vi "Acquisition Engine.vi"(0 "all channels":cluster{fxp<+/-,12,1>[]}[](array[cluster])=[{[0.0, 0.0, 0.0, 0.0, 0.0, 0.0, 0.0, 0.0, 0.0, 0.0, 0.0, 0.0, 0.0, 0.0, 0.0, 0.0]}, {[0.0, 0.0, 0.0, 0.0, 0.0, 0.0, 0.0, 0.0, 0.0, 0.0, 0.0, 0.0, 0.0, 0.0, 0.0, 0.0]}], 1 "delay buffer size":u16, 3 "DRAM FIFO v2 FPGA in":refnum<class "DRAM FIFO v2 FPGA.lvclass">, 5 "streaming control":T5={"flexrio.io.interleaving factor 0"=1, "flexrio.trigger.start.cfg 0"=0, "stream.num samples 0"=0, "stream.request state 0"=enum."Idle", "flexrio.stream.channels enabled 0"=0, "flexrio.buffer.delay.clocks 0"=0, "flexrio.buffer.delay.reset 0"=FALSE}, 7 "analog trigger":T4, 9 "ddc dsp":T3, 12 "User-defined Start Trigger - AI":bool) -> (4 "streaming indicators":T2, 6 "flexrio.dsp.ready 0":bool, 8 "start trigger to AO":bool)   [LabVIEW 2019, in "GettingStarted_5785_FPGA.lvlib"]
uses:
  GettingStarted_5785_FPGA.lvlib
  <instrlib>/_niInstr/Streaming/v1/FPGA/niInstr Streaming v1 FPGA.lvlib
  <instrlib>/FlexRIO/API/FPGA/v1/FlexRIO API FPGA v1.lvlib
  19501a50-0f1f-4491-a7af-f5ae35d08e33.vi
  <instrlib>/FlexRIO/API/FPGA/v1/Types/Start Trigger IO Resources.ctl
  <instrlib>/FlexRIO/API/FPGA/v1/IO/NI5785/FlexRIO 5785 FPGA v1.lvlib
  a554ad89-63b5-42fd-9d6e-5ac6acaa6c2d.vi
  <instrlib>/FlexRIO/DRAM FIFO/v2/FPGA/DRAM FIFO/DRAM FIFO v2 FPGA.lvclass
  <instrlib>/_niInstr/Data Formatting/v1/FPGA/niInstr Data Formatting v1 FPGA.lvlib
  77ebce0f-1de0-4771-a06a-aa915878c24f.vi
  517be193-3c03-40e8-8945-242d542ce425.vi
  fb9c666d-c109-4077-9c8d-4924348493cd.vi
  1d1eb1e1-a86c-4102-8133-5cf93c0bb657.vi
  dfb267dc-b7b8-4639-b659-0e0d8e0c4462.vi
  <vilib>/eio/EIONode/EIONode.xnode
  <vilib>/rvi/eio/common/nirviEmuTemplateMethod_errors.vi
  <instrlib>/_niInstr/Data Formatting/v1/FPGA/Private/Convert/U16 array to Boolean Array.vi
  <instrlib>/_niInstr/Streaming/v1/Common/Stream State.ctl
  <instrlib>/_niInstr/Streaming/v1/Common/niInstr Streaming v1 Common.lvlib
  DDC Cfg.ctl
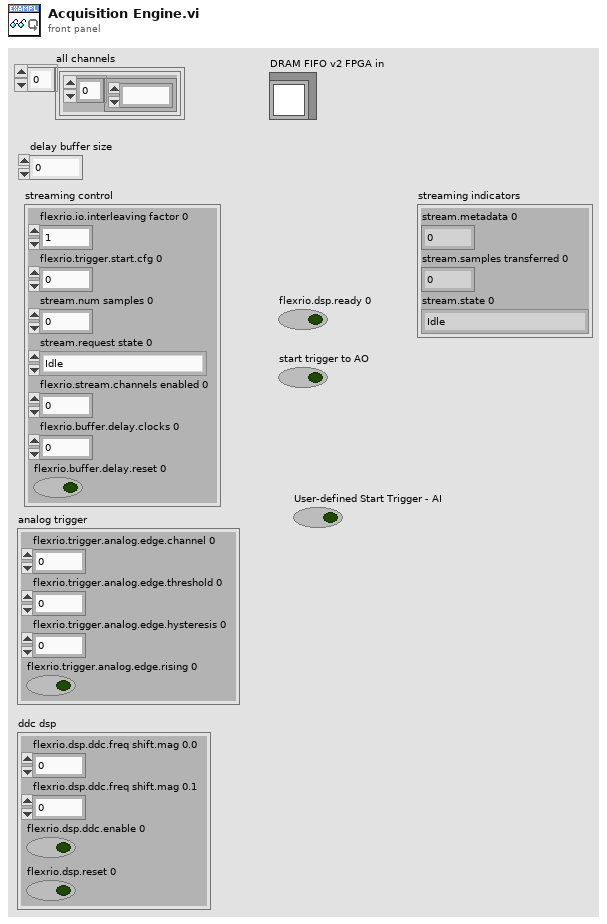
[diagram p1: front panel]
types:
  T1 = typedef "niInstr Streaming v1 Common.lvlib/Stream State.ctl" = enum8{"Idle", "Finite Transfer", "Continuous", "Done", "Error", "Not Ready", "Cancel"}
  T2 = cluster{"stream.metadata 0":u64, "stream.samples transferred 0":u64, "stream.state 0":T1}
  T3 = typedef "GettingStarted_5785_FPGA.lvlib/DDC Cfg.ctl" = cluster{"flexrio.dsp.ddc.freq shift.mag 0.0":fxp<+/-,48,0>, "flexrio.dsp.ddc.freq shift.mag 0.1":fxp<+/-,48,0>, "flexrio.dsp.ddc.enable 0":bool, "flexrio.dsp.reset 0":bool}
  T4 = cluster{"flexrio.trigger.analog.edge.channel 0":fxp<+,2,2>, "flexrio.trigger.analog.edge.threshold 0":fxp<+/-,32,1>, "flexrio.trigger.analog.edge.hysteresis 0":fxp<+/-,32,1>, "flexrio.trigger.analog.edge.rising 0":bool}
  T5 = cluster{"flexrio.io.interleaving factor 0":u16, "flexrio.trigger.start.cfg 0":u16, "stream.num samples 0":u64, "stream.request state 0":T1, "flexrio.stream.channels enabled 0":u64, "flexrio.buffer.delay.clocks 0":u16, "flexrio.buffer.delay.reset 0":bool}
  T6 = typedef "FlexRIO API FPGA v1.lvlib/Start Trigger IO Resources.ctl" = cluster{"start trigger":refnum<k21>, "started event":refnum<k21>, "start trigger for export":refnum<k21>, "start trigger for tclk":refnum<k21>}
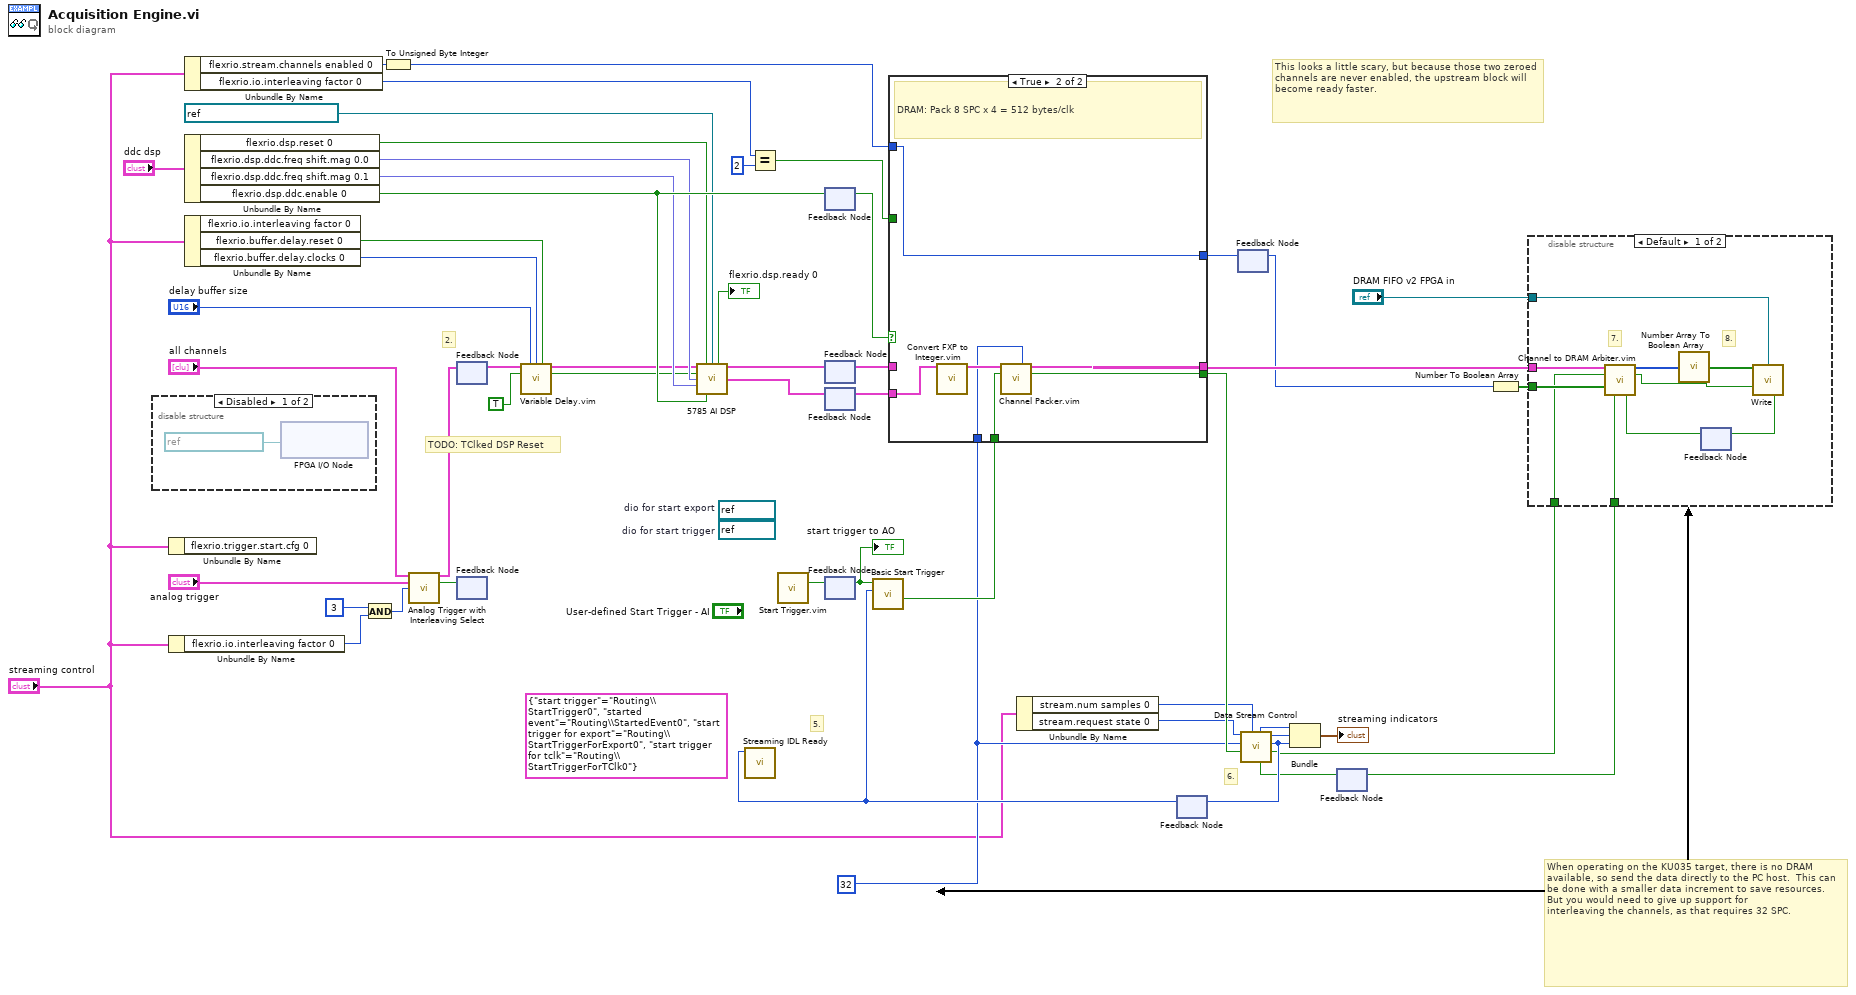
[diagram p0: block diagram]
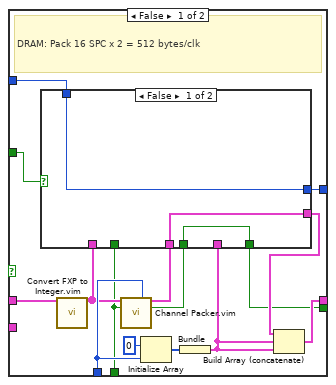
[diagram p3: hidden frame]
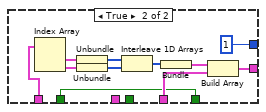
[diagram p4: hidden frame]
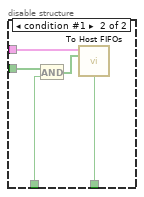
[diagram p5: hidden frame]
diagram:
  w11 = 32 ("output spc")
  (unwired) T6 {"start trigger"="Routing\\StartTrigger0", "started event"="Routing\\StartedEvent0", "start trigger for export"="Routing\\StartTriggerForExport0", "start trigger for tclk"="Routing\\StartTriggerForTClk0"} ("trigger io resources")
  (unwired) refnum<k21> "DIO 0"  # dio for start trigger
  (unwired) refnum<k21> "DIO 1"  # dio for start export
  # "TODO: TClked DSP Reset"
  # "When operating on the KU035 target, there is no DRAM available, so send the data directly to the PC host.  This can be done with a smaller data increment to save resources.  But you would need to give up support for\ninterleaving the channels, as that requires 32 SPC."
  # "This looks a little scary, but because those two zeroed channels are never enabled, the upstream block will become ready faster."
  # "5."
  # "2."
  # "6."
  n1 = disable-structure shown="Disabled" {
    frame Disabled {
      n2 = xnode "FPGA I/O Node"("FPGA I/O In"=refnum<k21> "Routing\\TClk") -> ()  [unwired: 2 out]
    }
    frame Enabled {
    }
  }
  n3 = Unbundle By Name("streaming control") -> ()  [unwired: 1 out]
  n4 = Unbundle By Name("streaming control") -> ("flexrio.io.interleaving factor 0"=w52:u16)
  n5 = Unbundle By Name("streaming control") -> ("flexrio.stream.channels enabled 0"=w6:u64, "flexrio.io.interleaving factor 0"=w7:u16)
  n6 = Unbundle By Name("ddc dsp") -> ("flexrio.dsp.reset 0"=w14:bool, "flexrio.dsp.ddc.freq shift.mag 0.0"=w46:fxp<+/-,48,0>, "flexrio.dsp.ddc.freq shift.mag 0.1"=w47:fxp<+/-,48,0>, "flexrio.dsp.ddc.enable 0"=w51:bool)
  n7 = Unbundle By Name("streaming control") -> ("flexrio.buffer.delay.reset 0"=w15:bool, "flexrio.buffer.delay.clocks 0"=w16:u16)  [unwired: 1 out]
  n8 = And(x=u16 3, y=w52) -> (x .and. y?=w17:u16)
  n9 = To Unsigned Byte Integer(number=w6) -> (unsigned 8bit integer=w3:u8)
  n10 = call "Analog Trigger with Interleaving Select.vi"("all channels"="all channels", "config"="analog trigger", "interleaving factor"=w17) -> ("all channels delayed out"=w2:cluster{fxp<+/-,12,1>[]}[], "triggered"=w24:bool)  [unwired: 11 in]
  n11 = feedback #1() -> (w1:cluster{fxp<+/-,12,1>[]}[])  [unwired: 1 in]
  n12 = feedback-in #1(w2) -> ()
  n13 = feedback #2() -> ()  [unwired: 2 in]
  n14 = feedback-in #2(w24) -> ()
  n15 = call "Variable Delay.vim"("Array in"=w1, "maximum delay"="delay buffer size", "delay"=w16, "reset"=w15, "data valid"=TRUE) -> ("Array out"=w34:cluster{fxp<+/-,12,1>[]}[], "data valid?"=w33:bool)  [unwired: 8 in, 1 out]
  n16 = call <instrlib>:"5785 AI DSP.vi"("all channels"=w34, "flexrio.dsp.reset 0"=w14, "clock x 2"=refnum<k21> "IO Socket\\Data Clock 2x", "input valid"=w33, "flexrio.dsp.ddc.freq shift.mag 0.0"=w46, "flexrio.dsp.ddc.freq shift.mag 0.1"=w47, "ddc enabled"=w51) -> ("flexrio.dsp.ready 0"=→"flexrio.dsp.ready 0":bool, "all channels no dsp"=w38:cluster{fxp<+/-,12,1>[]}[], "all channels with decimation"=w36:cluster{fxp<+/-,12,1>[]}[])  [unwired: 3 in, 3 out]
  n17 = Equal?(x=w7, y=u16 2 ("x")) -> (x = y?=w9:bool)
  n18 = call "Start Trigger.vim"() -> ("conditioned start trigger"=w26:bool)  [unwired: 13 in, 2 out]
  n19 = feedback #3() -> (w50:bool)  [unwired: 1 in]
  n20 = feedback-in #3(w51) -> ()
  n21 = feedback #4() -> (w43:cluster{fxp<+/-,12,1>[]}[])  [unwired: 1 in]
  n22 = feedback-in #4(w38) -> ()
  n23 = feedback #5() -> (w44:cluster{fxp<+/-,12,1>[]}[])  [unwired: 1 in]
  n24 = feedback-in #5(w36) -> ()
  n25 = feedback #6() -> (w49:bool)  [unwired: 1 in]
  "start trigger to AO" <- w49
  n26 = feedback-in #6(w26) -> ()
  n27 = Unbundle By Name("streaming control") -> ("stream.num samples 0"=w13:u64, "stream.request state 0"=w12:T1)
  n28 = feedback #7() -> (w18:T1)  [unwired: 1 in]
  n29 = call <instrlib>:"Streaming IDL Ready.vi"("stream.state"=w18) -> ()  [unwired: 10 in, 1 out]
  n30 = call <instrlib>:"Basic Start Trigger.vi"("stream.state"=w18, "start trigger"=w49) -> ("data valid"=w29:bool)  [unwired: 9 in]
  n31 = case shown="True" w50 {
    tunnel: w29 -> [w62 w88]
    tunnel: [w56 w87] -> w35
    tunnel: w44 -> [_ w86]
    tunnel: [w67 w85] -> w37
    tunnel: w43 -> [w68 _]
    tunnel: w11 -> [w64 w84]
    tunnel: w9 -> [w58 _]
    tunnel: w3 -> [w55 w83]
    tunnel: [w54 w83] -> w5
    frame False {
      # "DRAM: Pack 16 SPC x 2 = 512 bytes/clk"
      n32 = call "Convert FXP to Integer.vim"("Array in"=w68) -> ("Array"=w63:cluster{i16[]}[])  [unwired: 14 in]
      n33 = call "Channel Packer.vim"("Array in"=w63, "output spc"=w64, "data valid"=w62) -> ("Array out"=w61:cluster{i16[]}[], "full"=w60:bool)  [unwired: 11 in]
      n34 = Initialize Array(i16 0, w64) -> (w66:i16[])
      n35 = Bundle(w66) -> (w59:cluster{i16[]})  [unwired: 1 in]
      n36 = case shown="False" w58 {
        tunnel: w63 -> [_ w76]
        tunnel: w62 -> [_ w73]
        tunnel: w61 -> [w71 _]
        tunnel: w60 -> [w70 _]
        tunnel: w59 -> [_ w75]
        tunnel: [w71 w74] -> w57
        tunnel: [w70 w73] -> w56
        tunnel: w55 -> [w69 _]
        tunnel: [w69 u8 1] -> w54
        frame False {
        }
        frame True {
          n37 = Index Array(array=w76) -> (element #1=w77:cluster{i16[]}, element #2=w78:cluster{i16[]})  [unwired: 2 in]
          n38 = Unbundle(w77) -> (w79:i16[])
          n39 = Unbundle(w78) -> (w80:i16[])
          n40 = Interleave 1D Arrays(w79, w80) -> (w81:i16[])
          n41 = Bundle(w81) -> (w82:cluster{i16[]})  [unwired: 1 in]
          n42 = Build Array(w82, w75) -> (w74:cluster{i16[]}[])
        }
      }
      n43 = Build Array (concatenate)(w57, w59, w59) -> (w67:cluster{i16[]}[])
    }
    frame True {
      # "DRAM: Pack 8 SPC x 4 = 512 bytes/clk"
      n44 = call "Convert FXP to Integer.vim"("Array in"=w86) -> ("Array"=w89:cluster{i16[]}[])  [unwired: 14 in]
      n45 = call "Channel Packer.vim"("Array in"=w89, "output spc"=w84, "data valid"=w88) -> ("Array out"=w85:cluster{i16[]}[], "full"=w87:bool)  [unwired: 11 in]
    }
  }
  n46 = feedback-in #8(w5) -> ()
  n47 = feedback #8() -> (w4:u8)  [unwired: 1 in]
  n48 = feedback #9() -> (w23:bool)  [unwired: 1 in]
  n49 = call <instrlib>:"Data Stream Control.vi"("ready for input?"=w23, "stream.num samples 0"=w13, "data valid"=w35, "element count"=w11, "stream.request state 0"=w12) -> ("send data"=w20:bool, "stream.state 0"=w41:T1, "stream.samples transferred 0"=w40:u64, "stream.metadata 0"=w39:u64)  [unwired: 2 in, 1 out]
  n50 = feedback-in #7(w41) -> ()
  n51 = Bundle("stream.metadata 0"=w39, "stream.samples transferred 0"=w40, "stream.state 0"=w41) -> (→"streaming indicators":T2)  [unwired: 1 in]
  n52 = Number To Boolean Array(number=w4) -> (Boolean array=w19:bool[])
  n53 = disable-structure shown="Default" {
    disable-tunnel: w19 -> [w98 w102]
    disable-tunnel: w20 -> [w97 w103]
    disable-tunnel: "DRAM FIFO v2 FPGA in" -> [w94 _]
    disable-tunnel: [w92 w100] -> w22
    disable-tunnel: w37 -> [w91 w104]
    frame condition #0 (active) {
      # "8."
      # "7."
      n54 = feedback #10() -> (w93:bool)  [unwired: 1 in]
      n55 = call "Channel to DRAM Arbiter.vim"("channels in"=w91, "valid in"=w97, "channels enabled"=w98, "ready for output"=w93) -> ("data"=w99:i16[], "valid out"=w95:bool, "ready for input"=w92:bool)  [unwired: 9 in]
      n56 = call-poly <instrlib>:"Number Array To Boolean Array.vi"("data in"=w99) -> ("data out"=w90:bool[])  [unwired: 14 in]
      n57 = call <instrlib>:"Write.vi"("element"=w90, "DRAM FIFO ref in"=w94, "input valid"=w95) -> ("ready for input"=w96:bool)  [unwired: 12 in]
      n58 = feedback-in #10(w96) -> ()
    }
    frame condition #1 {
      n59 = And(x=w102, y=w103) -> (x .and. y?=w101:bool[])
      n60 = call "To Host FIFOs.vi"("data"=w104, "data valid"=w101) -> ("all ready for input"=w100:bool)  [unwired: 12 in, 1 out]
    }
  }
  n61 = feedback-in #9(w22) -> ()
